vi "Down Sampler 2-1.vi"(1 "stream in":T1) -> (0 "stream out":T1)   [LabVIEW 2023]
uses:
  <extravilib>/ChannelInstances/Stream-dbl/)Channel.ctl
  <extravilib>/ChannelInstances/Stream-dbl/Read With Abort.vi
  <extravilib>/ChannelInstances/Stream-dbl/Write With Abort.vi
  <extravilib>/ChannelInstances/Stream-dbl/EndpointRead.vi
  <extravilib>/ChannelInstances/Stream-dbl/Endpoint.vi
  <extravilib>/ChannelInstances/Stream-dbl/)Channel.vi
  <resource>/ChannelSupport/_ChannelSupport/WaitIfNeeded.vi
  <extravilib>/ChannelInstances/Stream-dbl.lvlib
panel:
  out "output value":dbl format="%.2f"
  out "input value":dbl format="%.2f"
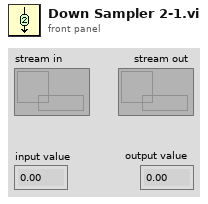
[diagram p1: front panel]
types:
  T1 = typedef "Stream-dbl.lvlib/)Channel.ctl" = refnum<queue>
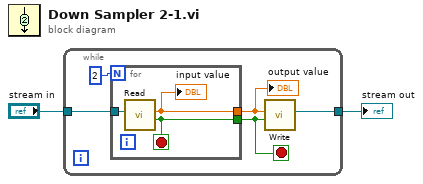
[diagram p0: block diagram]
diagram:
  n1 = while {
    tunnel: "stream in" -> [w5]
    tunnel: [w4] -> w1
    stop <- w3 stop-if-true
    n2 = for {
      N: 2 -> [_]
      tunnel: [w8] -> w3
      tunnel: [w9] -> w6
      tunnel: w5 -> [w10]
      stop <- w8 stop-if-true
      n3 = call <extravilib>:"Read.vi"("channel"=w10) -> ("last element?"=w8:bool, "element"=w9:dbl)  [unwired: 6 in, 3 out]
      "input value" <- w9
    }
    "output value" <- w6
    n4 = call <extravilib>:"Write.vi"("last element? (F)"=w3, "element"=w6) -> ("channel"=w4:T1)  [unwired: 7 in, 2 out]
  }
  "stream out" <- w1
